vi "IIR Cascade Filter PtbyPt Vec.vi"(2 "initialize":bool, 3 "IIR Filter Cluster":T1={"filter structure"=enum."IIR 2nd Order", "Reverse Coefficients"=[0.0, 0.0], "Forward Coefficients"=[1.0, 0.0, 0.0]}, 4 "Initial value":dbl[](array[numeric]) format="%0.2f", 5 "X":dbl[](array[numeric])=[0.0] format="%0.2f") -> (1 "Filtered X":dbl[](array[numeric]) format="%0.2f")   [LabVIEW 2013]
panel:
  # "Like the Labview standard non \"Vec\" VI except that X is a vector of multiple channels that are run through the same filter.  Also, on reset the initial state is computed differently so that it is as though the filter had been in steady-state with the current input, rather than whatever the Labview VI is trying to do.  We also only support second order sections, not fourth order (which Labview seems to only use for bandstop responses.)"
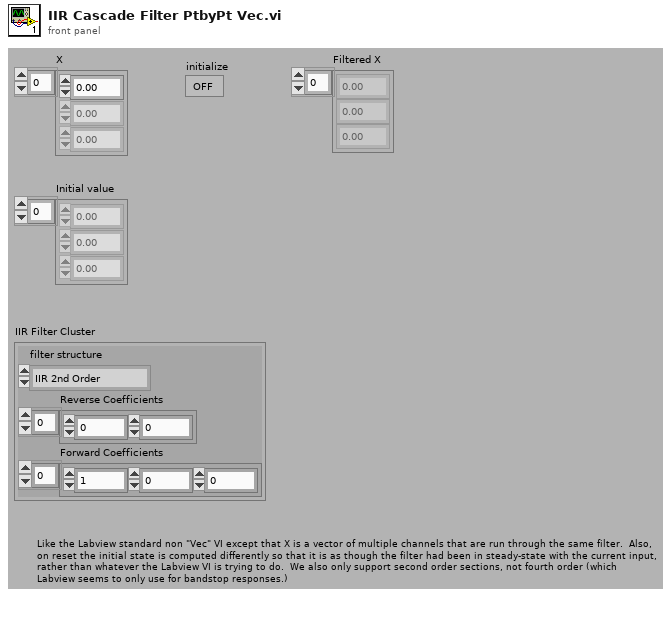
[diagram p1: front panel]
types:
  T1 = cluster{"filter structure":enum32{"IIR 2nd Order", "IIR 4th Order"}, "Reverse Coefficients":dbl[], "Forward Coefficients":dbl[]}
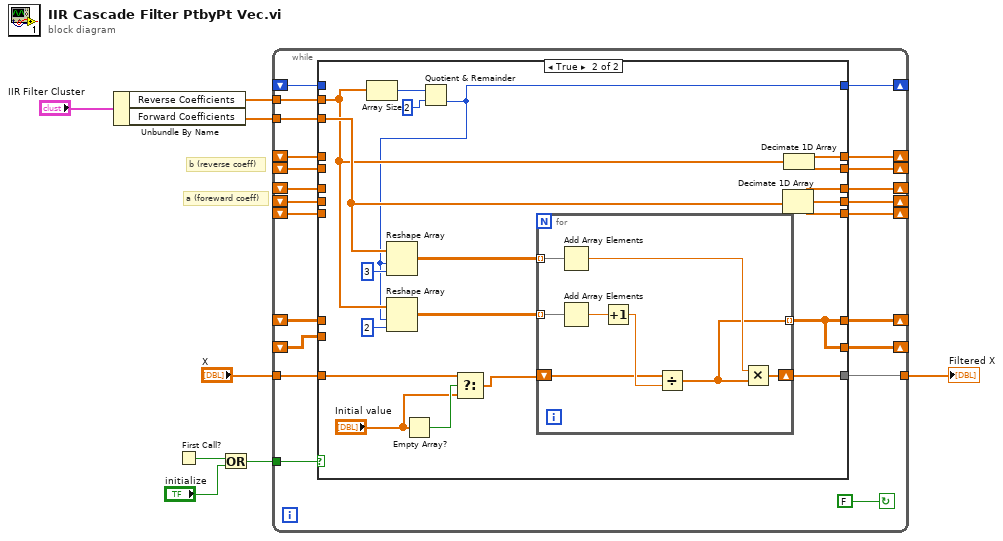
[diagram p0: block diagram]
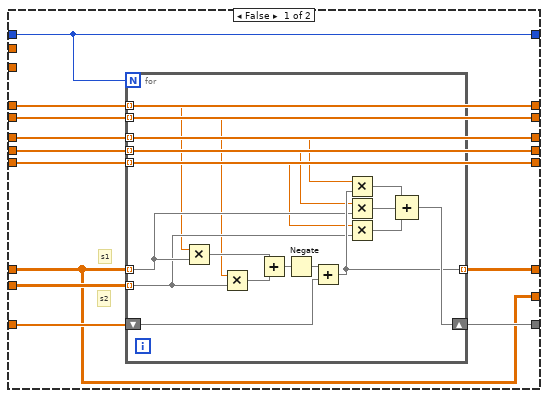
[diagram p2: hidden frame]
diagram:
  # "a (foreward coeff)"
  # "b (reverse coeff)"
  n1 = Unbundle By Name("IIR Filter Cluster") -> ("Reverse Coefficients"=w6:dbl[], "Forward Coefficients"=w7:dbl[])
  n2 = First Call?() -> (First Call?: T/F=w1:bool)
  n3 = Or(x=w1, y="initialize") -> (x .or. y?=w4:bool)
  n4 = while {
    tunnel: [w15] -> w5
    shift-left: _ -> [w16]
    shift-right: [w14] -> _
    shift-left: _ -> [w9]
    shift-right: [w19] -> _
    shift-left: _ -> [w20]
    shift-right: [w21] -> _
    shift-left: _ -> [w22]
    shift-right: [w23] -> _
    tunnel: "X" -> [w24]
    tunnel: w6 -> [w25]
    shift-left: _ -> [w26]
    shift-right: [w28] -> _
    shift-left: _ -> [w27]
    shift-right: [w29] -> _
    shift-left: _ -> [w17]
    shift-right: [w18] -> _
    tunnel: w7 -> [w30]
    tunnel: w4 -> [w12]
    shift-right: [w11] -> _
    shift-left: _ -> [w10]
    stop <- FALSE continue-if-true
    n5 = case shown="True" w12 {
      tunnel: w30 -> [_ w71]
      tunnel: [w39 w76] -> w29
      tunnel: [w38 w75] -> w28
      tunnel: w27 -> [w39 _]
      tunnel: w26 -> [w38 _]
      tunnel: w25 -> [_ w68]
      tunnel: w24 -> [w34 w62]
      tunnel: [w36 w77] -> w23
      tunnel: w22 -> [w36 _]
      tunnel: [w40 w74] -> w21
      tunnel: w20 -> [w40 _]
      tunnel: [w37 w78] -> w19
      tunnel: w9 -> [w37 _]
      tunnel: [w41 w63] -> w18
      tunnel: w17 -> [w41 _]
      tunnel: [w35 w65] -> w15
      tunnel: w16 -> [w32 _]
      tunnel: [w31 w64] -> w14
      tunnel: [w33 w64] -> w11
      tunnel: w10 -> [w31 _]
      frame False {
        # "s2"
        # "s1"
        n6 = for {
          N: w41 -> [_]
          tunnel: w31 -> [w48] mode=indexing
          tunnel: w32 -> [w47] mode=indexing
          tunnel: [w49] -> w33 mode=indexing
          shift-right: [w50] -> w35
          shift-left: w34 -> [w51]
          tunnel: w40 -> [w46] mode=indexing
          tunnel: w39 -> [w45] mode=indexing
          tunnel: w38 -> [w44] mode=indexing
          tunnel: w37 -> [w43] mode=indexing
          tunnel: w36 -> [w42] mode=indexing
          n7 = Multiply(x=w43, y=w48) -> (x*y=w58:dbl[])
          n8 = Multiply(x=w42, y=w47) -> (x*y=w57:dbl[])
          n9 = Add(x=w58, y=w57) -> (x+y=w56:dbl[])
          n10 = Negate(x=w56) -> (-x=w55:dbl[])
          n11 = Add(x=w55, y=w51) -> (x+y=w49:dbl[])
          n12 = Multiply(x=w46, y=w49) -> (x*y=w54:dbl[])
          n13 = Multiply(x=w45, y=w48) -> (x*y=w53:dbl[])
          n14 = Multiply(x=w44, y=w47) -> (x*y=w52:dbl[])
          n15 = Compound Arithmetic op=ADD(w54, w53, w52) -> (w50:dbl[])
        }
      }
      frame True {
        n16 = Array Size(array=w68) -> (size(s)=w73:i32)
        n17 = Empty Array?(array="Initial value") -> (empty?=w61:bool)
        n18 = Quotient & Remainder(x=w73, y=2) -> (floor(x/y)=w63:i32)  [unwired: 1 out]
        n19 = Reshape Array(w71, w63, 3 ("dimension size")) -> (w67:dbl[][])
        n20 = Reshape Array(w68, w63, 2 ("dimension size")) -> (w66:dbl[][])
        n21 = Select(t=w62, s=w61, f="Initial value") -> (s? t:f=w59:dbl[])
        n22 = for {
          tunnel: w67 -> [w85] mode=indexing
          tunnel: w66 -> [w84] mode=indexing
          shift-right: [w83] -> w65
          shift-left: w59 -> [w80]
          tunnel: [w79] -> w64 mode=indexing
          n23 = Add Array Elements(numeric array=w85) -> (sum=w82:dbl)
          n24 = Add Array Elements(numeric array=w84) -> (sum=w86:dbl)
          n25 = Increment(x=w86) -> (x+1=w81:dbl)
          n26 = Divide(x=w80, y=w81) -> (x/y=w79:dbl[])
          n27 = Multiply(x=w82, y=w79) -> (x*y=w83:dbl[])
        }
        n28 = Decimate 1D Array(w71) -> (w74:dbl[], w76:dbl[], w75:dbl[])
        n29 = Decimate 1D Array(w68) -> (w78:dbl[], w77:dbl[])
      }
    }
  }
  "Filtered X" <- w5
